vi "triggerIRQInstruction.vi"(8 "error in (no error)":errorcluster, 9 "Subnet":u8, 10 "ModbusBuffer in":refnum<class "ModbusBuffer.lvclass">, 11 "ILCCommunications in":refnum<class "ILCCommunications.lvclass">) -> (0 "error out":errorcluster, 2 "ModbusBuffer out":refnum<class "ModbusBuffer.lvclass">, 3 "ILCCommunications out":refnum<class "ILCCommunications.lvclass">)   [LabVIEW 2016, in "ILCCommunications.lvclass"]
uses:
  ILCCommunications.lvclass
  Common_RT_Modbus/ModbusBuffer/ModbusBuffer.lvclass
  Common_RT_Modbus/ModbusBuffer/ModbusBuffer.lvclass/ModbusBuffer.ctl
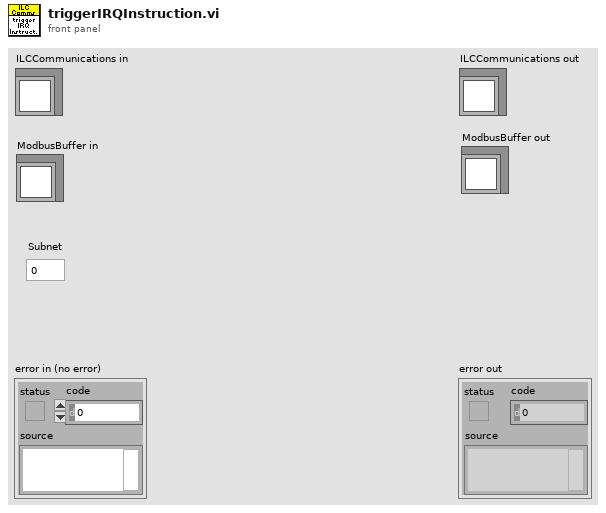
[diagram p1: front panel]
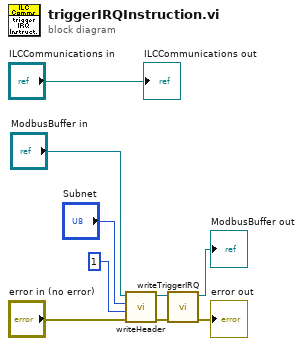
[diagram p0: block diagram]
diagram:
  n1 = call "writeHeader.vi"("error in (no error)"="error in (no error)", "Length"=u16 1, "Subnet"="Subnet", "ModbusBuffer in"="ModbusBuffer in") -> ("error out"=w8:errorcluster, "ModbusBuffer out"=w7:refnum<class "ModbusBuffer.lvclass">)  [unwired: 6 in]
  n2 = call "writeTriggerIRQ.vi"("error in (no error)"=w8, "ModbusBuffer in"=w7) -> ("error out"=→"error out":errorcluster, "ModbusBuffer out"=→"ModbusBuffer out":refnum<class "ModbusBuffer.lvclass">)  [unwired: 8 in]
  "ILCCommunications out" <- "ILCCommunications in"
